vi "idPassword.vi"() -> ()   [LabVIEW 2020]
panel:
  in  "Amount":string
  out "s? t:f":string
  out "output":string
  in  "PIN":string
  in  "User Name":string
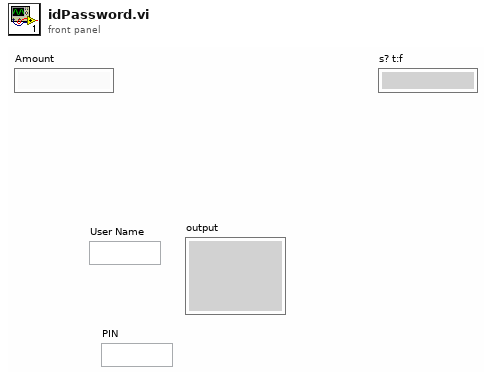
[diagram p1: front panel]
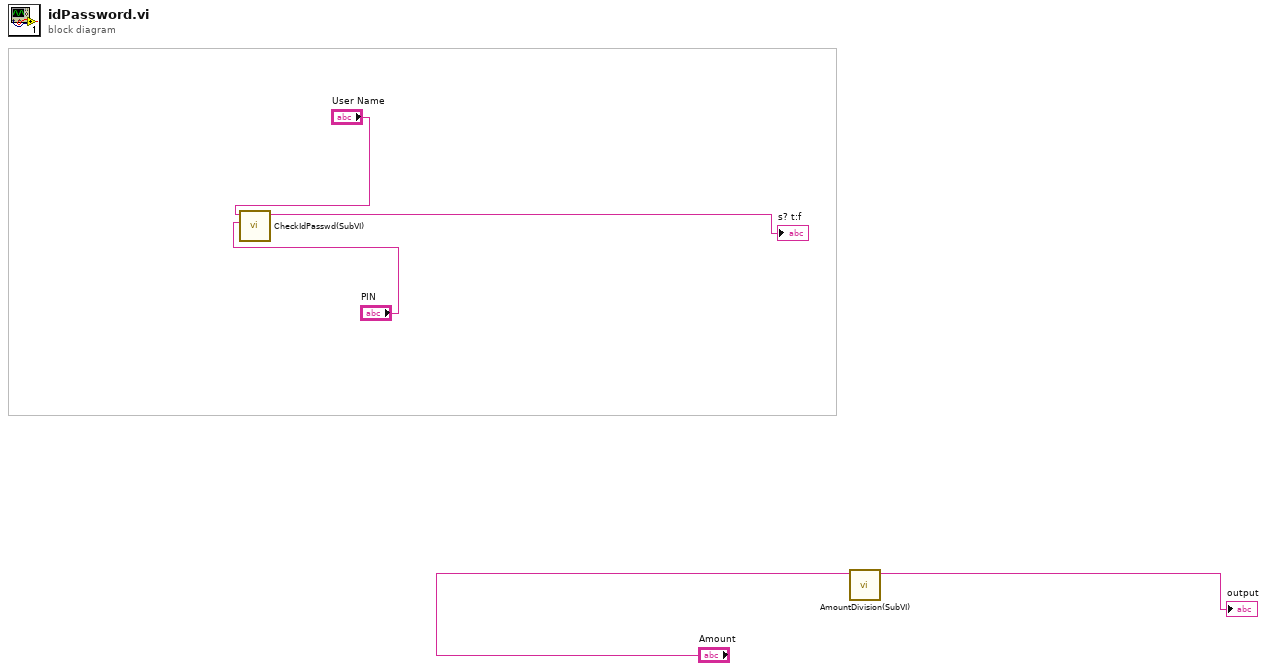
[diagram p0: block diagram]
diagram:
  n1 = call "CheckIdPasswd(SubVI).vi"("PIN"="PIN", "User Name"="User Name") -> ("s? t:f"=→"s? t:f":string)  [unwired: 9 in]
  n2 = call "AmountDivision(SubVI).vi"("Amount"="Amount") -> ("output"=→"output":string)  [unwired: 10 in]
